vi "PH_SHS_Analysis_Calibrator.set modified data.vi"(0 "i ref in":refnum<vi>, 2 "i attribute":T1={"GUI Refs"={"Available Cams"=refnum, "OK"=refnum, "Skip"=refnum, "Repeat"=refnum, "Cancel"=refnum, "Dialog"=refnum, "Enough Images?"=refnum}, "Cam instances"=[], "Status"={"#"=0, "Data calculated"=FALSE, "Wanted #"=0}, "IMAQ Image Array"=[], "Pixel Size [µm]"=6.7, "MLA Pitch [µm]"=200.0, "Method"=enum."automatic", "Enough Images?"=FALSE, "SHS Reference Result"={"Reference"=[], "Lens Array Pitch [px]"=0.0}, "Calculation Error"={"status"=FALSE, "code"=0, "source"=""}}, 5 "error in (no error)":errorcluster) -> (14 "i ref out":refnum<vi>, 19 "error out":errorcluster)   [LabVIEW 2014, in "PH_SHS_Analysis_Calibrator.lvlib"]
doc: "Writes the data into the attribute of an object. Then, the attribute dara are unlocked using the \"release\" method. Prior to calling THIS method, the attribute data must have been locked using the methods \"lock\" or \"get data to modify\".\n\n\nLicense Agreement for this software:\n\nCopyright (C)\nGesellschaft für Schwerionenforschung, GSI\nPlanckstr. 1\n64291 Darmstadt\nGermany\n\nContact: D.Beck@gsi.de \n\nThis program is free software; you can redistribute it and/or modify it under the terms of the GNU General Public License as published by the Free Software Foundation; either version 2 of the license, or (at your option) any later version.\n\nThis program is distributed in the hope that it will be useful, but WITHOUT ANY WARRANTY; without even the implied warranty of MERCHANTABILITY or FITNESS FOR A PARTICULAR PURPOSE. See the GNU General License for more details (http://www.gnu.org).\n\nGesellschaft für Schwerionenforschung, GSI\nPlanckstr. 1, 64291 Darmstadt, Germany\nFor all questions and ideas contact: M.Richter@gsi.de, H.Brand@gsi.de or D.Beck@gsi.de.\nLast update: 17-JUN-2004"
uses:
  PH_SHS_Analysis_Calibrator.lvlib
  PH_SHS_Analysis_Calibrator.i attribute.ctl
  <vilib>/vision/Image Controls.llb/IMAQ Image.ctl
  User/Eisenbarth/SHS_v4/SHS_Common/SHSReference.ctl
  User/Eisenbarth/SHS_v4/SHS_Common/ReferencePoint.ctl
  User/Eisenbarth/SHS_v4/SHS_Common/Rectangle.ctl
  User/Eisenbarth/SHS_v4/SHS_Common/Point.ctl
  CSCore/CSObj/CSObj.lvlib
  User/Eisenbarth/SHS_v4/SHS_Common/SHS_Common.lvlib
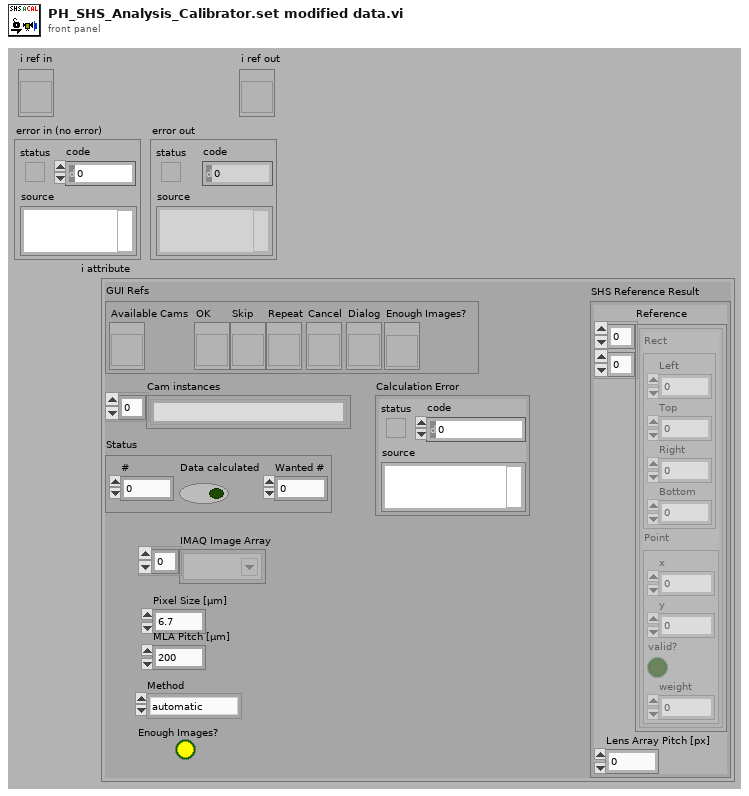
[diagram p1: front panel]
types:
  T1 = typedef "PH_SHS_Analysis_Calibrator.lvlib/PH_SHS_Analysis_Calibrator.i attribute.ctl" = cluster{"GUI Refs":cluster{"Available Cams":refnum<vi>, "OK":refnum<vi>, "Skip":refnum<vi>, "Repeat":refnum<vi>, "Cancel":refnum<vi>, "Dialog":refnum<vi>, "Enough Images?":refnum<vi>}, "Cam instances":string[], "Status":cluster{"#":i32, "Data calculated":bool, "Wanted #":i32}, "IMAQ Image Array":T2[], "Pixel Size [µm]":dbl, "MLA Pitch [µm]":dbl, "Method":enum16{"automatic", "manual"}, "Enough Images?":bool, "SHS Reference Result":T3, "Calculation Error":errorcluster}
  T2 = typedef "IMAQ Image.ctl" = refnum<image>
  T3 = typedef "SHS_Common.lvlib/SHSReference.ctl" = cluster{"Reference":T4[][], "Lens Array Pitch [px]":dbl}
  T4 = typedef "SHS_Common.lvlib/ReferencePoint.ctl" = cluster{"Rect":T5, "Point":T6}
  T5 = typedef "SHS_Common.lvlib/Rectangle.ctl" = cluster{"Left":i32, "Top":i32, "Right":i32, "Bottom":i32}
  T6 = typedef "SHS_Common.lvlib/Point.ctl" = cluster{"x":dbl, "y":dbl, "valid?":bool, "weight":dbl}
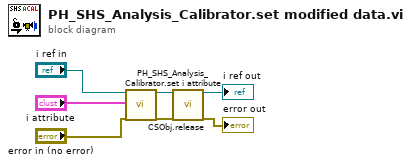
[diagram p0: block diagram]
diagram:
  n1 = call "PH_SHS_Analysis_Calibrator.set i attribute.vi"("i ref in"="i ref in", "i attribute"="i attribute", "error in (no error)"="error in (no error)") -> ("i ref out"=w4:refnum<vi>, "error out"=w3:errorcluster)  [unwired: 15 in]
  n2 = call "CSObj.release.vi"("i ref in"=w4, "error in (no error)"=w3) -> ("i ref out"=→"i ref out":refnum<vi>, "error out"=→"error out":errorcluster)  [unwired: 16 in]
